vi "create_error_message.vi"(8 "error in (no error)":errorcluster, 10 "Error Message":errorcluster, 11 "role":string) -> (0 "error out":errorcluster, 3 "message_text out":refnum<class "message_text.lvclass">)   [LabVIEW 2020, in "message_text.lvclass"]
uses:
  message_text.lvclass
  message.ctl
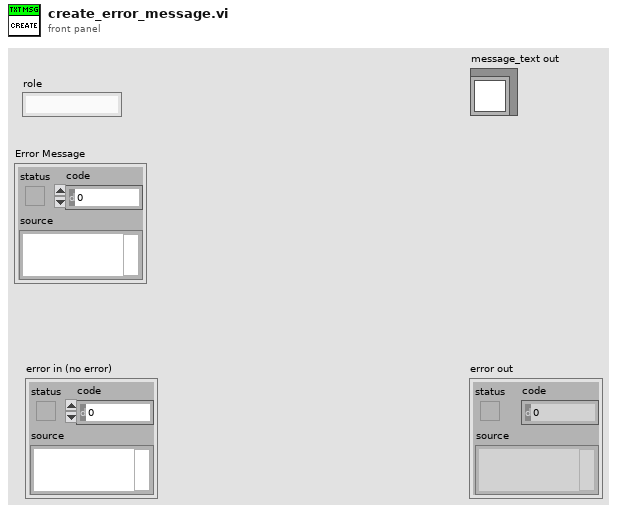
[diagram p1: front panel]
types:
  T1 = typedef "message_text.lvclass/message.ctl" = cluster{"role":string, "content":string[]}
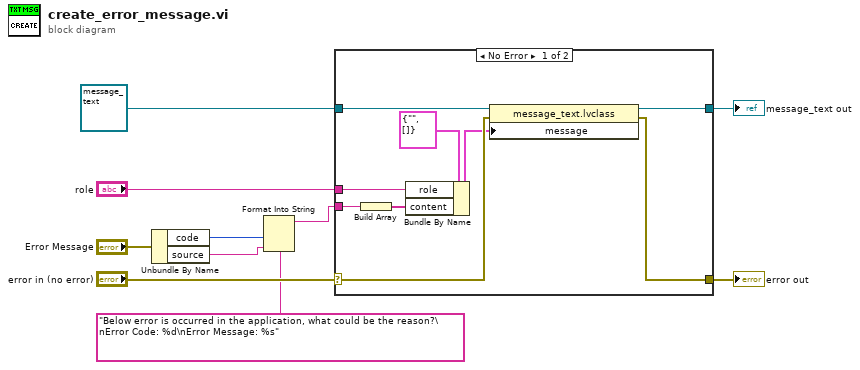
[diagram p0: block diagram]
diagram:
  n1 = Unbundle By Name("Error Message") -> ("code"=w4:i32, "source"=w3:string)
  n2 = Format Into String(format string="Below error is occurred in the application, what could be the reason?\nError Code: %d\nError Message: %s", w4, w3) -> (resulting string=w2:string)  [unwired: 2 in, 1 out]
  n3 = case shown="No Error" "error in (no error)" {
    selector: "error in (no error)" -> [w17 w21]
    tunnel: [w16 w21] -> w9
    tunnel: [w18 w20] -> w7
    tunnel: refnum<class "message_text.lvclass"> refnum ("message_text in") -> [w19 w20]
    tunnel: w2 -> [w13 _]
    tunnel: "role" -> [w12 _]
    frame No Error {
      n4 = Build Array(w13) -> (w11:string[])
      n5 = Bundle By Name(cluster=T1 {"role"="", "content"=[]} ("message"), "role"=w12, "content"=w11) -> (w14:T1)
      n6 = property class="message_text.lvclass"(reference=w19, error in=w17, "message"=w14) -> (reference out=w18:refnum<class "message_text.lvclass">, error out=w16:errorcluster)
    }
    frame Error {
    }
  }
  "error out" <- w9
  "message_text out" <- w7
